vi "Write Header Information.vi"(8 "error in (no error)":errorcluster, 11 "Save Image in":refnum<class "Save Image.lvclass">) -> (0 "error out":errorcluster, 3 "Save Image out":refnum<class "Save Image.lvclass">)   [LabVIEW 2018, in "Save Image.lvclass"]
uses:
  Save Image.lvclass
  <userlib>/atmcd32d.llb/Shutter_mode typedef.ctl
  <userlib>/atmcd32d.llb/ReadMode_mode typedef.ctl
  <userlib>/atmcd32d.llb/AcquisitionMode_mode typedef.ctl
  Save Image.lvclass/Save Image.ctl
  Interface/Interface.lvclass
  TCS_ACS/TCS_ACS.lvclass
  Simulated_Header/Simulated_Header.lvclass
panel:
  out "CCD Config":T4
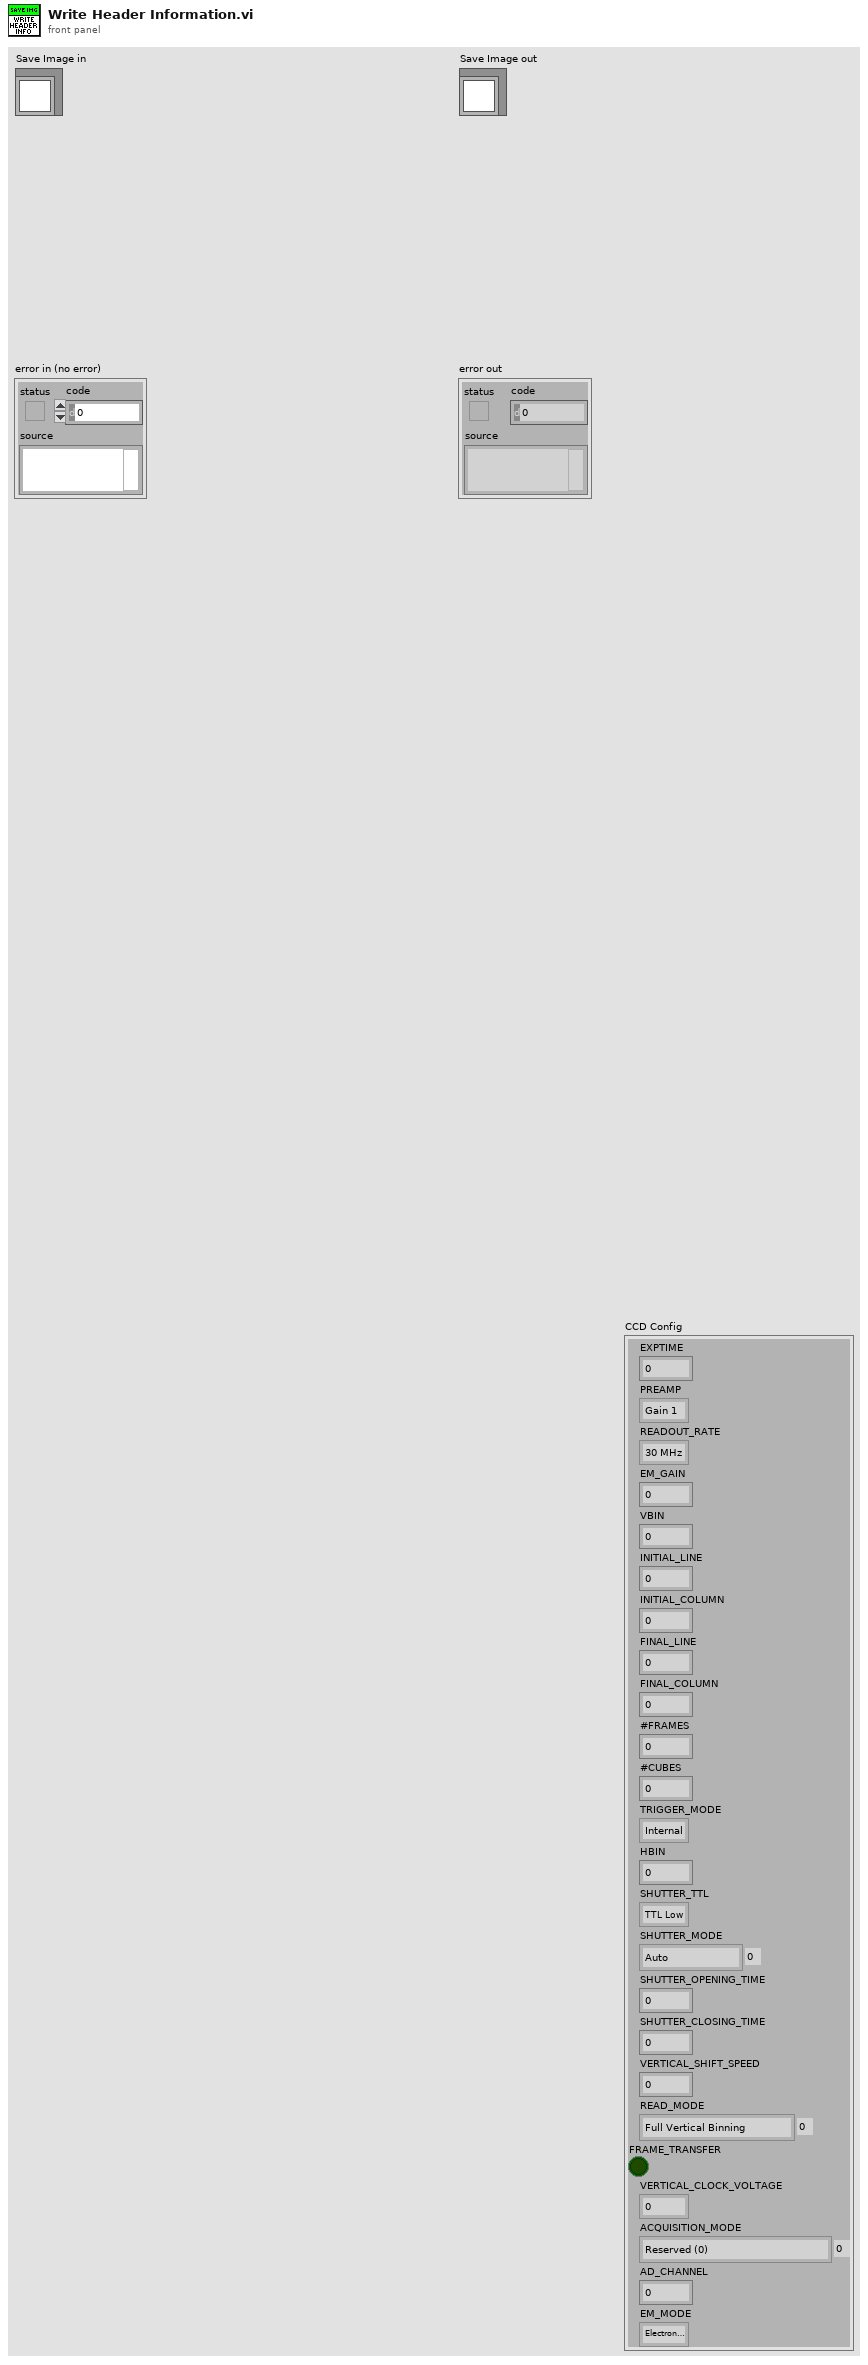
[diagram p1: front panel]
types:
  T1 = typedef "Shutter_mode typedef.ctl" = enum16{"Auto", "Open", "Close", "N/A (3)", "Open FVB Series", "Open Any Series"}
  T2 = typedef "ReadMode_mode typedef.ctl" = enum16{"Full Vertical Binning", "Multi-Track", "Random-Track", "Single-Track", "Image"}
  T3 = typedef "AcquisitionMode_mode typedef.ctl" = enum16{"Reserved (0)", "Single Scan", "Accumulate", "Kinetics", "Fast Kinetics", "Run Till Abort", "Reserved (6)", "Reserved (7)", "Reserved (8)", "Time Delayed Integration"}
  T4 = cluster{"EXPTIME":sgl, "PREAMP":enum16{"Gain 1", "Gain 2"}, "READOUT_RATE":enum16{"30 MHz", "20 MHz", "10 MHz", "1 MHz"}, "EM_GAIN":u16, "VBIN":u16, "INITIAL_LINE":u16, "INITIAL_COLUMN":u16, "FINAL_LINE":u16, "FINAL_COLUMN":u16, "#FRAMES":u32, "#CUBES":u32, "TRIGGER_MODE":enum16{"Internal", "External", "N/A", "N/A_1", "N/A_2", "N/A_3", "External Start"}, "HBIN":u16, "SHUTTER_TTL":enum16{"TTL Low", "TTL High"}, "SHUTTER_MODE":T1, "SHUTTER_OPENING_TIME":u16, "SHUTTER_CLOSING_TIME":u16, "VERTICAL_SHIFT_SPEED":u16, "READ_MODE":T2, "FRAME_TRANSFER":bool, "VERTICAL_CLOCK_VOLTAGE":enum16{"0", "+1", "+2", "+3", "+4"}, "ACQUISITION_MODE":T3, "AD_CHANNEL":u16, "EM_MODE":enum16{"Electron Multiplying", "Conventional"}}
  T5 = cluster{"OBJ":string, "RA":string, "DEC":string, "EPOCH":dbl, "AIRMASS":dbl, "JD":dbl, "SD":string, "HA":string, "DATEOBS":string, "FOCUS":string, "WS_DEFAULT":string, "TEMP":string, "BAR":string, "HUM":string, "FILTER":string}
  T6 = cluster{"CUBE_EXPOSURE_TIME":sgl, "CUBES_DONE":u16, "LAST_IMAGE_NAME":string, "DISK_SPACE":u16, "FRAMES_DONE":u16, "CCD_STATUS":string, "CURRENT_TEMPERATURE":i16, "TEMPERATURE_STATUS":string, "FRAME_EXPOSURE_TIME":u16, "CCD_ON_OFF":bool, "SERIAL_NUMBER":u16, "ACQUIRING":bool}
  T7 = cluster{"FILENAME":cluster{"Name":string, "Value":string, "Comment":string}, "OBSERVER":cluster{"Name":string, "Value":string, "Comment":string}, "PROGRID":cluster{"Name":string, "Value":string, "Comment":string}, "OBJECT":cluster{"Name":string, "Value":string, "Comment":string}, "NIGHTDIR":cluster{"Name":string, "Value":string, "Comment":string}, "CHANNEL":cluster{"Name":string, "Value":string, "Comment":string}, "INSTRUME":cluster{"Name":string, "Value":string, "Comment":string}, "NEXPSEQ":cluster{"Name":string, "Value":u16, "Comment":string}, "SEQINDEX":cluster{"Name":string, "Value":u16, "Comment":string}, "OBSTYPE":cluster{"Name":string, "Value":string, "Comment":string}, "READMOD":cluster{"Name":string, "Value":string, "Comment":string}, "READMODE":cluster{"Name":string, "Value":string, "Comment":string}, "ACQMODE":cluster{"Name":string, "Value":string, "Comment":string}, "PREAMP":cluster{"Name":string, "Value":string, "Comment":string}, "READOUT":cluster{"Name":string, "Value":string, "Comment":string}, "VSHIFT":cluster{"Name":string, "Value":string, "Comment":string}, "TRIGGER":cluster{"Name":string, "Value":string, "Comment":string}, "EMMODE":cluster{"Name":string, "Value":string, "Comment":string}, "EMGAIN":cluster{"Name":string, "Value":u16, "Comment":string}, "VBIN":cluster{"Name":string, "Value":u16, "Comment":string}, "HBIN":cluster{"Name":string, "Value":u16, "Comment":string}, "INITLIN":cluster{"Name":string, "Value":u16, "Comment":string}, "INITCOL":cluster{"Name":string, "Value":u16, "Comment":string}, "FINALLIN":cluster{"Name":string, "Value":u16, "Comment":string}, "FINALCOL":cluster{"Name":string, "Value":u16, "Comment":string}, "KSERLEN":cluster{"Name":string, "Value":u16, "Comment":string}, "SHUTTER":cluster{"Name":string, "Value":string, "Comment":string}, "OPENSHT":cluster{"Name":string, "Value":u16, "Comment":string}, "CLOSESHT":cluster{"Name":string, "Value":u16, "Comment":string}, "DATE":cluster{"Name":string, "Value":string, "Comment":string}, "GAIN":cluster{"Name":string, "Value":dbl, "Comment":string}, "GAINERR":cluster{"Name":string, "Value":dbl, "Comment":string}, "RDNOISE":cluster{"Name":string, "Value":dbl, "Comment":string}, "RNOISERR":cluster{"Name":string, "Value":dbl, "Comment":string}, "SKYFIBER":cluster{"Name":string, "Value":string, "Comment":string}, "CALFIBER":cluster{"Name":string, "Value":string, "Comment":string}, "UTDATE":cluster{"Name":string, "Value":string, "Comment":string}, "LOCTIME":cluster{"Name":string, "Value":string, "Comment":string}, "MJD":cluster{"Name":string, "Value":dbl, "Comment":string}, "OBSLON":cluster{"Name":string, "Value":string, "Comment":string}, "OBSLAT":cluster{"Name":string, "Value":string, "Comment":string}, "OBSALT":cluster{"Name":string, "Value":dbl, "Comment":string}, "EXPTIME":cluster{"Name":string, "Value":dbl, "Comment":string}, "TELRA":cluster{"Name":string, "Value":string, "Comment":string}, "TELDEC":cluster{"Name":string, "Value":string, "Comment":string}, "RA":cluster{"Name":string, "Value":string, "Comment":string}, "DEC":cluster{"Name":string, "Value":string, "Comment":string}, "RA_DEG":cluster{"Name":string, "Value":dbl, "Comment":string}, "DEC_DEG":cluster{"Name":string, "Value":dbl, "Comment":string}, "EPOCH":cluster{"Name":string, "Value":dbl, "Comment":string}, "HA":cluster{"Name":string, "Value":string, "Comment":string}, "HAD":cluster{"Name":string, "Value":dbl, "Comment":string}, "AIRMASS":cluster{"Name":string, "Value":dbl, "Comment":string}, "AMSTART":cluster{"Name":string, "Value":dbl, "Comment":string}, "AMEND":cluster{"Name":string, "Value":dbl, "Comment":string}, "XOFFSET":cluster{"Name":string, "Value":dbl, "Comment":string}, "YOFFSET":cluster{"Name":string, "Value":dbl, "Comment":string}, "PA":cluster{"Name":string, "Value":dbl, "Comment":string}, "CAMFOC":cluster{"Name":string, "Value":string, "Comment":string}, "TELFOC":cluster{"Name":string, "Value":dbl, "Comment":string}, "TCSUT":cluster{"Name":string, "Value":string, "Comment":string}, "TCSST":cluster{"Name":string, "Value":string, "Comment":string}, "MOONDIST":cluster{"Name":string, "Value":dbl, "Comment":string}, "MOONALT":cluster{"Name":string, "Value":dbl, "Comment":string}, "MOONPHAS":cluster{"Name":string, "Value":string, "Comment":string}, "ADC":cluster{"Name":string, "Value":string, "Comment":string}, "ADCSPEED":cluster{"Name":string, "Value":dbl, "Comment":string}, "CALMIRR":cluster{"Name":string, "Value":string, "Comment":string}, "GUIDING":cluster{"Name":string, "Value":string, "Comment":string}, "GUIDTEXP":cluster{"Name":string, "Value":dbl, "Comment":string}, "GUIDFREQ":cluster{"Name":string, "Value":dbl, "Comment":string}, "GUIDOBJX":cluster{"Name":string, "Value":dbl, "Comment":string}, "GUIDOBJY":cluster{"Name":string, "Value":dbl, "Comment":string}, "AVGYCORR":cluster{"Name":string, "Value":dbl, "Comment":string}, "AVGXCORR":cluster{"Name":string, "Value":dbl, "Comment":string}, "GFOCUS":cluster{"Name":string, "Value":dbl, "Comment":string}, "THARLAMP":cluster{"Name":string, "Value":string, "Comment":string}, "HALLAMP":cluster{"Name":string, "Value":string, "Comment":string}, "AGITATOR":cluster{"Name":string, "Value":string, "Comment":string}, "THARMIRR":cluster{"Name":string, "Value":string, "Comment":string}, "DSTATUS":cluster{"Name":string, "Value":string, "Comment":string}, "DPOS":cluster{"Name":string, "Value":dbl, "Comment":string}, "DTEMP":cluster{"Name":string, "Value":dbl, "Comment":string}, "DHUM":cluster{"Name":string, "Value":string, "Comment":string}, "DLAMP":cluster{"Name":string, "Value":string, "Comment":string}, "DFLAT":cluster{"Name":string, "Value":string, "Comment":string}, "TEMPEXT":cluster{"Name":string, "Value":string, "Comment":string}, "PRESSURE":cluster{"Name":string, "Value":string, "Comment":string}, "HUMIDITY":cluster{"Name":string, "Value":string, "Comment":string}, "WINDDIR":cluster{"Name":string, "Value":string, "Comment":string}, "WINSPEED":cluster{"Name":string, "Value":dbl, "Comment":string}, "SHTTTL":cluster{"Name":string, "Value":string, "Comment":string}, "COOLER":cluster{"Name":string, "Value":string, "Comment":string}, "TEMP":cluster{"Name":string, "Value":u16, "Comment":string}, "TEMPST":cluster{"Name":string, "Value":string, "Comment":string}, "SERN":cluster{"Name":string, "Value":u16, "Comment":string}, "COMMENT":cluster{"Name":string, "Value":string, "Comment":string}, "SIMPLE":cluster{"Name":string, "Value":string, "Comment":string}, "BITPIX":cluster{"Name":string, "Value":u16, "Comment":string}, "NAXIS":cluster{"Name":string, "Value":u16, "Comment":string}, "EXTEND":cluster{"Name":string, "Value":string, "Comment":string}, "FRAME_T":cluster{"Name":string, "Value":string, "Comment":string}, "VCLOCK":cluster{"Name":string, "Value":string, "Comment":string}, "ADCHNNL":cluster{"Name":string, "Value":u16, "Comment":string}, "JD":cluster{"Name":string, "Value":dbl, "Comment":string}, "SD":cluster{"Name":string, "Value":string, "Comment":string}, "FILTER":cluster{"Name":string, "Value":string, "Comment":string}}
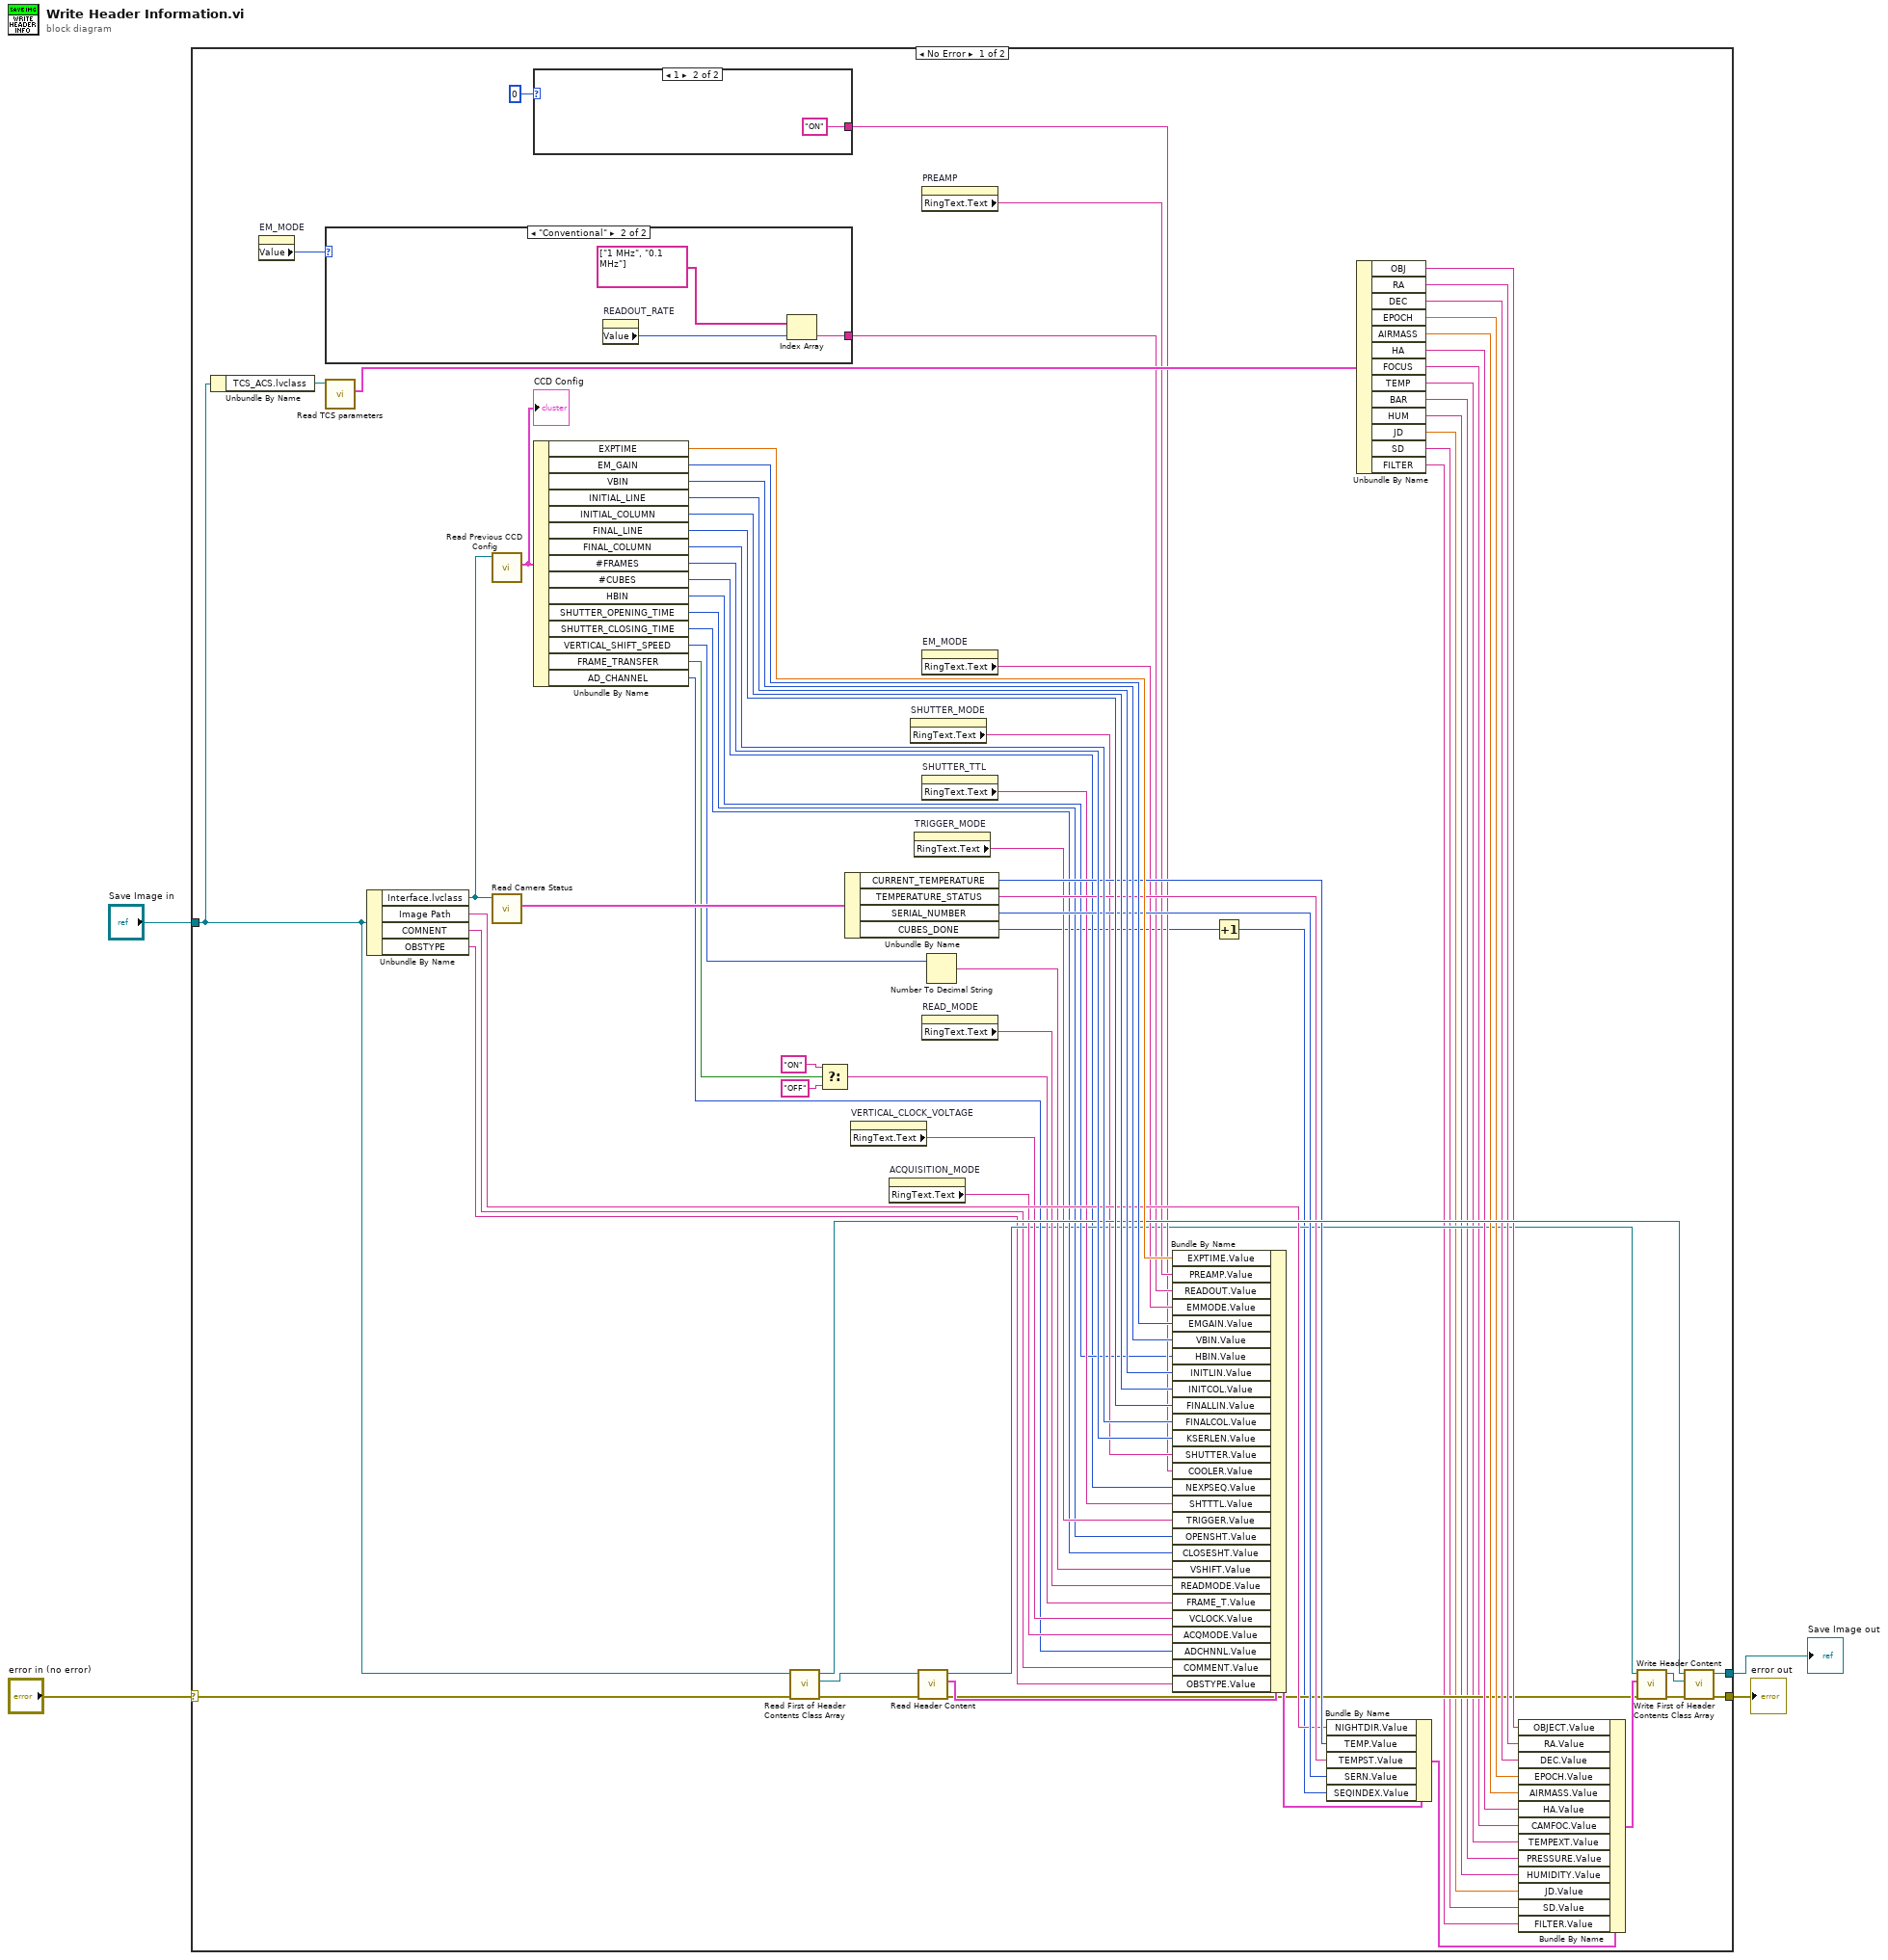
[diagram p0: block diagram]
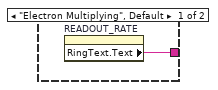
[diagram p2: hidden frame]
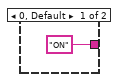
[diagram p3: hidden frame]
diagram:
  n1 = case shown="No Error" "error in (no error)" {
    selector: "error in (no error)" -> [w68 w83]
    tunnel: [w67 w83] -> w3
    tunnel: [w66 w84] -> w1
    tunnel: "Save Image in" -> [w58 w84]
    frame No Error {
      n2 = Unbundle By Name(w58) -> ("TCS_ACS.lvclass"=w57:refnum<class "TCS_ACS.lvclass">)
      n3 = property on="EM_MODE" class="Enum (strict)"() -> ("Value"=w14:enum16{"Electron Multiplying", "Conventional"})  [unwired: 2 in, 2 out]
      n4 = case shown="\"Conventional\"" w14 {
        tunnel: [w77 w78] -> w46
        frame "Electron Multiplying", Default {
          n5 = property on="READOUT_RATE" class="Enum (strict)"() -> ("RingText.Text"=w77:string)  [unwired: 2 in, 2 out]
        }
        frame "Conventional" {
          n6 = property on="READOUT_RATE" class="Enum (strict)"() -> ("Value"=w80:enum16{"30 MHz", "20 MHz", "10 MHz", "1 MHz"})  [unwired: 2 in, 2 out]
          n7 = Index Array(array=string[] ["1 MHz", "0.1 MHz"], index=w80) -> (element=w78:string)
        }
      }
      n8 = call "Read TCS parameters.vi"("TCS_ACS in"=w57) -> ("TCS parameters"=w55:T5)  [unwired: 8 in, 2 out]
      n9 = Unbundle By Name(w58) -> ("Interface.lvclass"=w19:refnum<class "Interface.lvclass">, "Image Path"=w48:string, "COMNENT"=w6:string, "OBSTYPE"=w5:string)
      n10 = call "Read Previous CCD Config.vi"("Interface in"=w19) -> ("Previous CCD Config"=w18:T4)  [unwired: 8 in, 2 out]
      "CCD Config" <- w18
      n11 = call "Read Camera Status.vi"("Interface in"=w19) -> ("Camera Status"=w64:T6)  [unwired: 8 in, 2 out]
      n12 = case shown="1" u8 0 ("Shutter Mode") {
        tunnel: ["ON" "ON"] -> w43
        frame 0, Default {
        }
        frame 1 {
        }
      }
      n13 = Unbundle By Name(w18) -> ("EXPTIME"=w76:sgl, "EM_GAIN"=w75:u16, "VBIN"=w74:u16, "INITIAL_LINE"=w73:u16, "INITIAL_COLUMN"=w72:u16, "FINAL_LINE"=w71:u16, "FINAL_COLUMN"=w70:u16, "#FRAMES"=w69:u32, "#CUBES"=w17:u32, "HBIN"=w40:u16, "SHUTTER_OPENING_TIME"=w39:u16, "SHUTTER_CLOSING_TIME"=w38:u16, "VERTICAL_SHIFT_SPEED"=w36:u16, "FRAME_TRANSFER"=w32:bool, "AD_CHANNEL"=w28:u16)
      n14 = call "Read First of Header Contents Class Array.vi"("error in (no error)"=w68, "Save Image in"=w58) -> ("error out"=w26:errorcluster, "Simulated_Header.lvclass"=w27:refnum<class "Simulated_Header.lvclass">, "Save Image out"=w65:refnum<class "Save Image.lvclass">)  [unwired: 7 in]
      n15 = Select(t="ON", s=w32, f="OFF") -> (s? t:f=w31:string)
      n16 = Unbundle By Name(w64) -> ("CURRENT_TEMPERATURE"=w63:i16, "TEMPERATURE_STATUS"=w60:string, "SERIAL_NUMBER"=w62:u16, "CUBES_DONE"=w16:u16)
      n17 = property on="VERTICAL_CLOCK_VOLTAGE" class="Enum (strict)"() -> ("RingText.Text"=w30:string)  [unwired: 2 in, 2 out]
      n18 = property on="ACQUISITION_MODE" class="Enum (strict)"() -> ("RingText.Text"=w29:string)  [unwired: 2 in, 2 out]
      n19 = property on="SHUTTER_MODE" class="Enum (strict)"() -> ("RingText.Text"=w44:string)  [unwired: 2 in, 2 out]
      n20 = property on="TRIGGER_MODE" class="Enum (strict)"() -> ("RingText.Text"=w41:string)  [unwired: 2 in, 2 out]
      n21 = call "Read Header Content.vi"("error in (no error)"=w26, "Simulated_Header in"=w27) -> ("error out"=w21:errorcluster, "Header Content"=w25:T7, "Simulated_Header out"=w20:refnum<class "Simulated_Header.lvclass">)  [unwired: 7 in]
      n22 = property on="PREAMP" class="Enum (strict)"() -> ("RingText.Text"=w47:string)  [unwired: 2 in, 2 out]
      n23 = property on="EM_MODE" class="Enum (strict)"() -> ("RingText.Text"=w45:string)  [unwired: 2 in, 2 out]
      n24 = property on="SHUTTER_TTL" class="Enum (strict)"() -> ("RingText.Text"=w42:string)  [unwired: 2 in, 2 out]
      n25 = property on="READ_MODE" class="Enum (strict)"() -> ("RingText.Text"=w35:string)  [unwired: 2 in, 2 out]
      n26 = Number To Decimal String(number=w36) -> (decimal integer string=w37:string)  [unwired: 1 in]
      n27 = Bundle By Name(cluster=w25, "EXPTIME.Value"=w76, "PREAMP.Value"=w47, "READOUT.Value"=w46, "EMMODE.Value"=w45, "EMGAIN.Value"=w75, "VBIN.Value"=w74, "HBIN.Value"=w40, "INITLIN.Value"=w73, "INITCOL.Value"=w72, "FINALLIN.Value"=w71, "FINALCOL.Value"=w70, "KSERLEN.Value"=w69, "SHUTTER.Value"=w44, "COOLER.Value"=w43, "NEXPSEQ.Value"=w17, "SHTTTL.Value"=w42, "TRIGGER.Value"=w41, "OPENSHT.Value"=w39, "CLOSESHT.Value"=w38, "VSHIFT.Value"=w37, "READMODE.Value"=w35, "FRAME_T.Value"=w31, "VCLOCK.Value"=w30, "ACQMODE.Value"=w29, "ADCHNNL.Value"=w28, "COMMENT.Value"=w6, "OBSTYPE.Value"=w5) -> (w59:T7)
      n28 = Increment(x=w16) -> (x+1=w15:u16)
      n29 = Bundle By Name(cluster=w59, "NIGHTDIR.Value"=w48, "TEMP.Value"=w63, "TEMPST.Value"=w60, "SERN.Value"=w62, "SEQINDEX.Value"=w15) -> (w56:T7)
      n30 = Unbundle By Name(w55) -> ("OBJ"=w54:string, "RA"=w53:string, "DEC"=w52:string, "EPOCH"=w51:dbl, "AIRMASS"=w50:dbl, "HA"=w49:string, "FOCUS"=w13:string, "TEMP"=w12:string, "BAR"=w11:string, "HUM"=w10:string, "JD"=w9:dbl, "SD"=w8:string, "FILTER"=w7:string)
      n31 = Bundle By Name(cluster=w56, "OBJECT.Value"=w54, "RA.Value"=w53, "DEC.Value"=w52, "EPOCH.Value"=w51, "AIRMASS.Value"=w50, "HA.Value"=w49, "CAMFOC.Value"=w13, "TEMPEXT.Value"=w12, "PRESSURE.Value"=w11, "HUMIDITY.Value"=w10, "JD.Value"=w9, "SD.Value"=w8, "FILTER.Value"=w7) -> (w24:T7)
      n32 = call "Write Header Content.vi"("error in (no error)"=w21, "Header Content"=w24, "Simulated_Header in"=w20) -> ("error out"=w22:errorcluster, "Simulated_Header out"=w23:refnum<class "Simulated_Header.lvclass">)  [unwired: 7 in]
      n33 = call "Write First of Header Contents Class Array.vi"("error in (no error)"=w22, "Simulated_Header.lvclass"=w23, "Save Image in"=w65) -> ("error out"=w67:errorcluster, "Save Image out"=w66:refnum<class "Save Image.lvclass">)  [unwired: 7 in]
    }
    frame Error {
    }
  }
  "error out" <- w3
  "Save Image out" <- w1
